vi "Send Trigger.vi"(8 "error in (no error)":errorcluster, 11 "NI PXI Trigger in":refnum<class "NI PXI Trigger.lvclass">) -> (0 "error out":errorcluster, 3 "NI PXI Trigger out":refnum<class "NI PXI Trigger.lvclass">)   [LabVIEW 2020, in "NI DAQmx.lvlib" / "NI PXI Trigger.lvclass"]
uses:
  NI PXI Trigger.lvclass
  NI PXI Trigger.lvclass/NI PXI Trigger.ctl
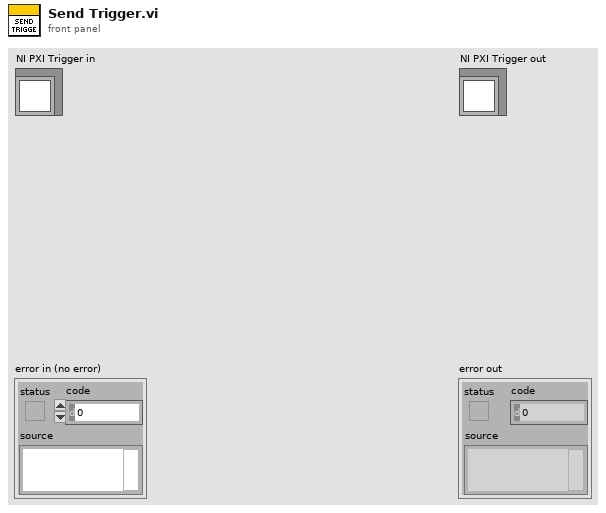
[diagram p1: front panel]
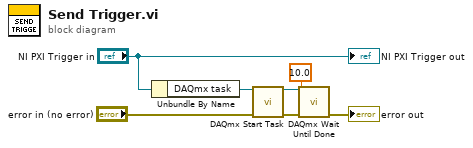
[diagram p0: block diagram]
diagram:
  n1 = Unbundle By Name("NI PXI Trigger in") -> ("DAQmx task"=w1:refnum<k21>)
  n2 = call <vilib>:"DAQmx Start Task.vi"("task/channels in"=w1, "error in"="error in (no error)") -> ("task out"=w7:refnum<k21>, "error out"=w3:errorcluster)  [unwired: 12 in]
  n3 = call <vilib>:"DAQmx Wait Until Done.vi"("task/channels in"=w7, "timeout (sec)"=10.0, "error in"=w3) -> ("error out"=→"error out":errorcluster)  [unwired: 11 in, 1 out]
  "NI PXI Trigger out" <- "NI PXI Trigger in"
